vi "Save DUT Information.vi"(8 "error in (no error)":errorcluster, 10 "DUT Info":T1, 11 "Formatter in":refnum<class "Formatter.lvclass">) -> (0 "error out":errorcluster, 3 "Formatter out":refnum<class "Formatter.lvclass">)   [LabVIEW 2015, in "Formatter.lvclass"]
doc: "This VI will save the DUT Information to the permanent report"
uses:
  Formatter.lvclass
  Report Information/DUT Information.ctl
  Report Information/Report Information.lvclass
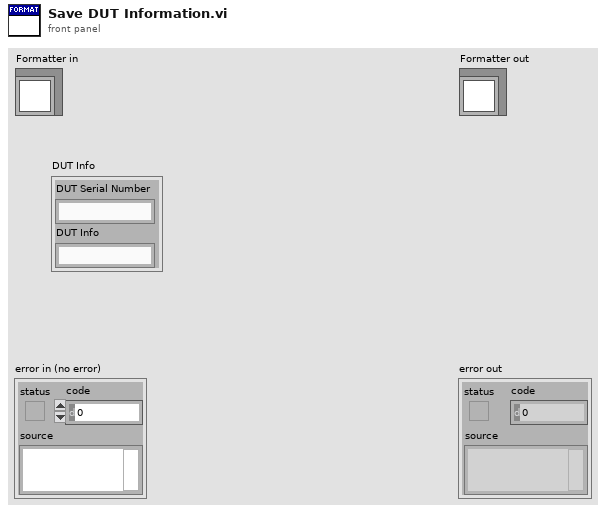
[diagram p1: front panel]
types:
  T1 = typedef "Report Information.lvclass/DUT Information.ctl" = cluster{"DUT Serial Number":string, "DUT Info":string}
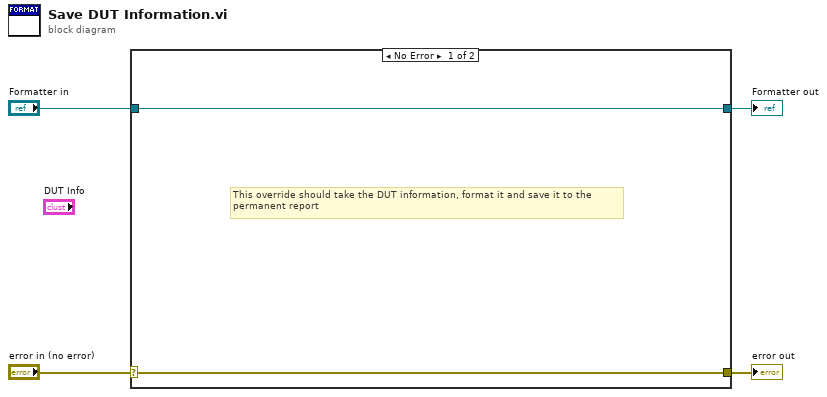
[diagram p0: block diagram]
diagram:
  n1 = case shown="No Error" "error in (no error)" {
    selector: "error in (no error)" -> [w5 w8]
    tunnel: [w5 w8] -> w3
    tunnel: [w6 w7] -> w1
    tunnel: "Formatter in" -> [w6 w7]
    frame No Error {
      # "This override should take the DUT information, format it and save it to the\npermanent report"
    }
    frame Error {
    }
  }
  "error out" <- w3
  "Formatter out" <- w1
